vi "Registry FGV.vi"(7 "State (Get Logger)":T2(ring)=enum."Get Logger", 8 "error in (no error)":errorcluster, 9 "Debug Level in":T1, 10 "Sink(s)":refnum<class "Sink.lvclass">[](array[class]), 11 "Name":string) -> (0 "error out":errorcluster, 1 "Debug Level out":T1=enum."DEBUG", 2 "Sinks":refnum<class "Sink.lvclass">[](array[class]), 3 "Logger out":refnum<class "Logger.lvclass">)   [LabVIEW 2020, in "LV Log.lvlib"]
uses:
  LV Log.lvlib
  Logger/Logger.lvclass
  Sinks/Sink/Sink.lvclass
  Type Defs/Debug Level.ctl
  Registry/Registry.lvclass
  Registry/Registry.lvclass/Registry.ctl
  <vilib>/ErrorRing/Error Ring.xnode
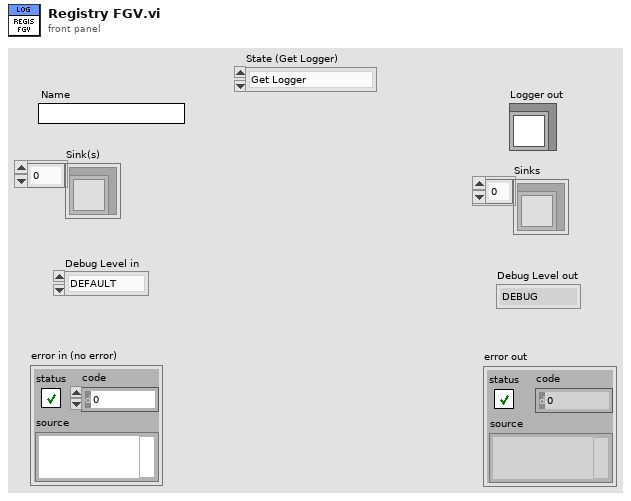
[diagram p1: front panel]
types:
  T1 = typedef "LV Log.lvlib/Debug Level.ctl" = enum16{"DEFAULT", "DEBUG", "INFO", "WARN", "ERROR", "FATAL"}
  T2 = enum16{"Init", "Get Logger", "Register Sink", "Set Global Debug Level", "Get Sinks", "Get Global Debug Level", "Register Logger"}
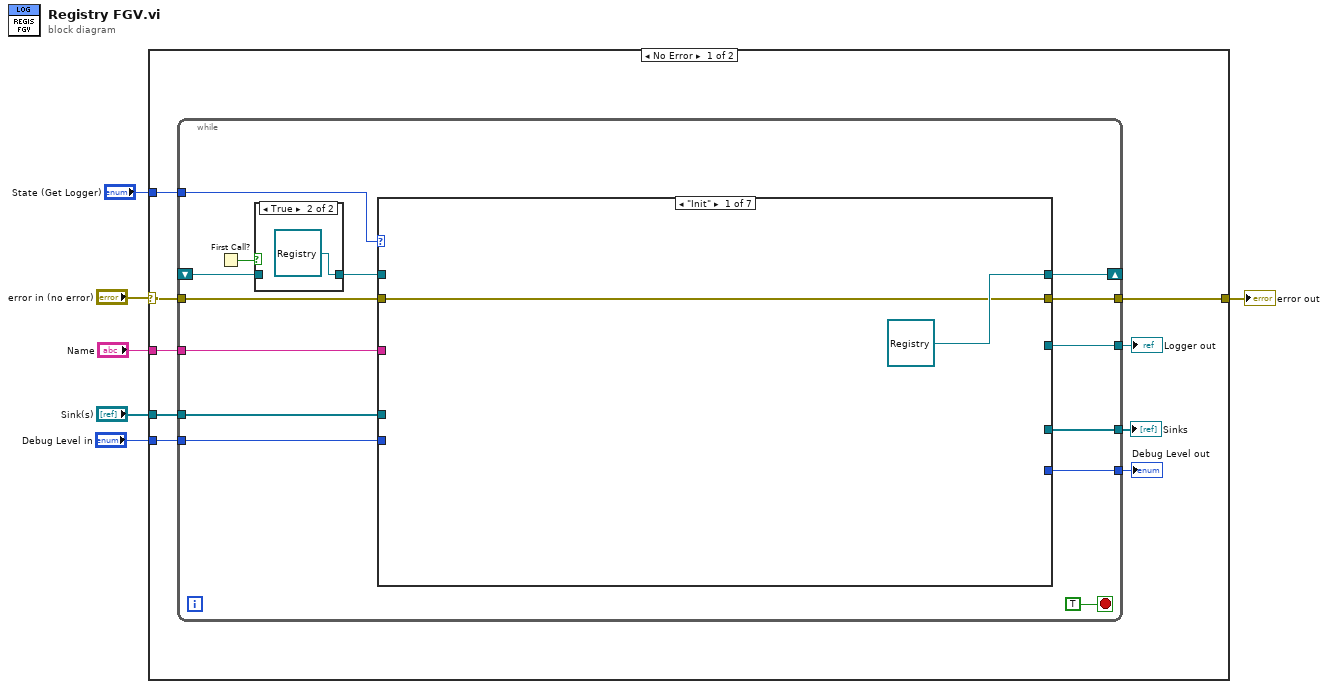
[diagram p0: block diagram]
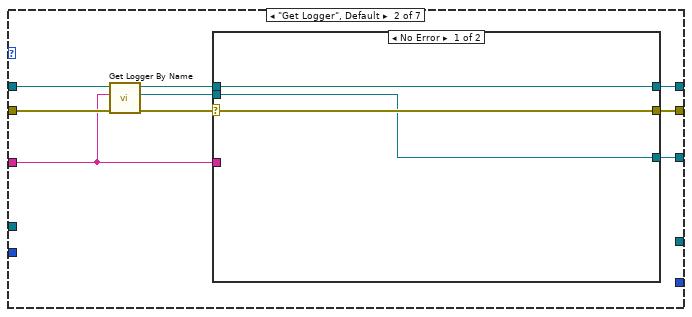
[diagram p3: hidden frame]
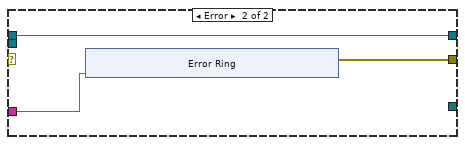
[diagram p4: hidden frame]
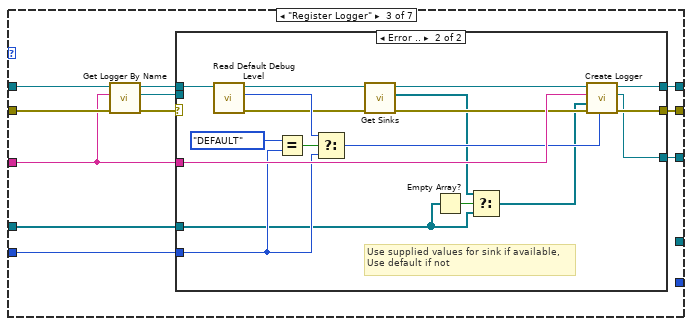
[diagram p5: hidden frame]
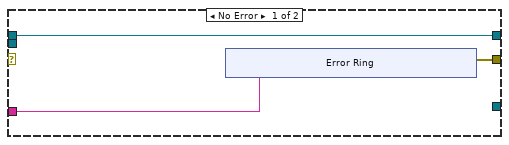
[diagram p6: hidden frame]
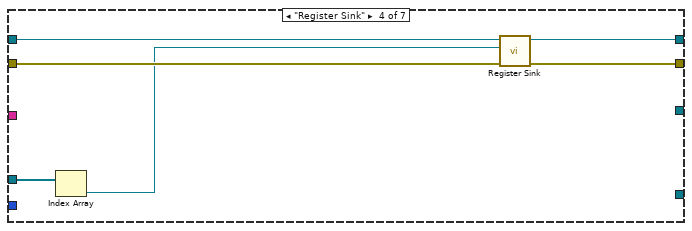
[diagram p7: hidden frame]
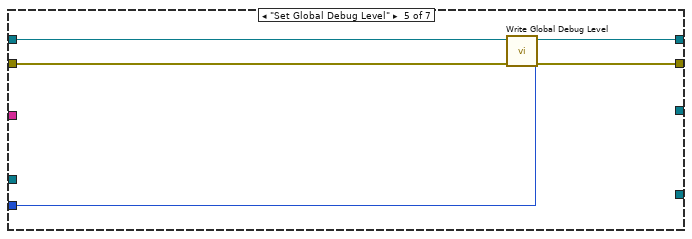
[diagram p8: hidden frame]
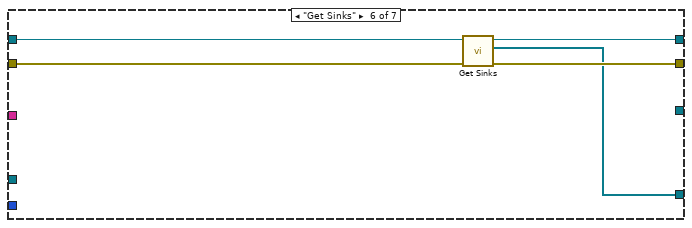
[diagram p9: hidden frame]
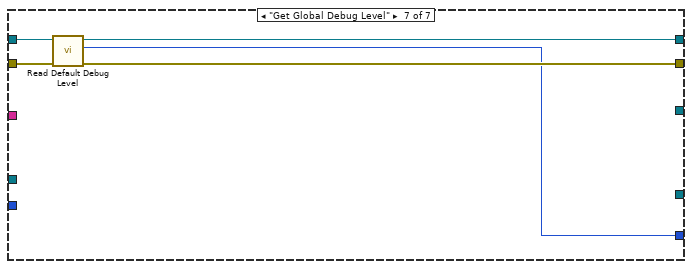
[diagram p10: hidden frame]
diagram:
  n1 = case shown="No Error" "error in (no error)" {
    selector: "error in (no error)" -> [w13 w112]
    tunnel: "State (Get Logger)" -> [w15 _]
    tunnel: "Name" -> [w14 _]
    tunnel: [w12 w112] -> w3
    tunnel: "Sink(s)" -> [w10 _]
    tunnel: "Debug Level in" -> [w8 _]
    frame No Error {
      n2 = while {
        shift-right: [w28] -> _
        shift-left: _ -> [w20]
        tunnel: w15 -> [w27]
        tunnel: w14 -> [w26]
        tunnel: w13 -> [w25]
        tunnel: [w24] -> w12
        tunnel: [w23] -> w11
        tunnel: w10 -> [w22]
        tunnel: [w21] -> w9
        tunnel: w8 -> [w17]
        tunnel: [w16] -> w7
        stop <- TRUE stop-if-true
        n3 = First Call?() -> (First Call?: T/F=w18:bool)
        n4 = case shown="True" w18 {
          tunnel: w20 -> [w30 _]
          tunnel: [w30 refnum<class "Registry.lvclass"> refnum ("LV Logging.lvlib:Registry.lvclass")] -> w19
          frame False {
          }
          frame True {
          }
        }
        n5 = case shown="\"Init\"" w27 {
          tunnel: [refnum<class "Registry.lvclass"> refnum ("LV Logging.lvlib:Registry.lvclass") w40 w62 w94 w100 w103 w109] -> w28
          tunnel: w26 -> [_ w35 w57 _ _ _ _]
          tunnel: w19 -> [_ w42 w64 w95 w101 w105 w111]
          tunnel: w25 -> [w32 w37 w59 w96 w99 w106 w110]
          tunnel: [w32 w36 w58 w93 w98 w104 w108] -> w24
          tunnel: [_ w34 w56 _ _ _ _] -> w23
          tunnel: w22 -> [_ _ w55 w92 _ _ _]
          tunnel: [_ _ _ _ _ w102 _] -> w21
          tunnel: w17 -> [_ _ w54 _ w97 _ _]
          tunnel: [_ _ _ _ _ _ w107] -> w16
          frame "Init" {
          }
          frame "Get Logger", Default {
            n6 = call "Get Logger By Name.vi"("error in (no error)"=w37, "Name"=w35, "Registry in"=w42) -> ("error out"=w39:errorcluster, "Logger"=w38:refnum<class "Logger.lvclass">, "Registry out"=w41:refnum<class "Registry.lvclass">)  [unwired: 6 in]
            n7 = case shown="No Error" w39 {
              selector: w39 -> [w44 _]
              tunnel: w41 -> [w45 w48]
              tunnel: [w45 w48] -> w40
              tunnel: w38 -> [w43 _]
              tunnel: [w44 w47] -> w36
              tunnel: w35 -> [_ w46]
              tunnel: [w43 _] -> w34
              frame No Error {
              }
              frame Error {
                n8 = xnode "Error Ring"("parameter 0"=w46) -> ("error out"=w47:errorcluster)
              }
            }
          }
          frame "Register Logger" {
            n9 = call "Get Logger By Name.vi"("error in (no error)"=w59, "Name"=w57, "Registry in"=w64) -> ("error out"=w61:errorcluster, "Logger"=w60:refnum<class "Logger.lvclass">, "Registry out"=w63:refnum<class "Registry.lvclass">)  [unwired: 6 in]
            n10 = case shown="Error .." w61 {
              tunnel: w63 -> [w67 w82]
              tunnel: [w67 w90] -> w62
              tunnel: w60 -> [_ _]
              tunnel: [w66 w89] -> w58
              tunnel: w57 -> [w65 w88]
              tunnel: [_ w87] -> w56
              tunnel: w55 -> [_ w74]
              tunnel: w54 -> [_ w84]
              frame No Error {
                n11 = xnode "Error Ring"("parameter 0"=w65) -> ("error out"=w66:errorcluster)
              }
              frame Error {
                # "Use supplied values for sink if available,\nUse default if not"
                n12 = call "Read Default Debug Level.vi"("Registry in"=w82) -> ("error out"=w78:errorcluster, "Debug Level"=w81:T1, "Registry out"=w80:refnum<class "Registry.lvclass">)  [unwired: 8 in]
                n13 = Equal?(x=Debug_Level."DEFAULT", y=w84) -> (x = y?=w85:bool)
                n14 = Select(t=w81, s=w85, f=w84) -> (s? t:f=w83:T1)
                n15 = call "Get Sinks.vi"("error in (no error)"=w78, "Registry in"=w80) -> ("error out"=w77:errorcluster, "Sinks"=w75:refnum<class "Sink.lvclass">[], "Registry out"=w79:refnum<class "Registry.lvclass">)  [unwired: 7 in]
                n16 = Empty Array?(array=w74) -> (empty?=w76:bool)
                n17 = Select(t=w75, s=w76, f=w74) -> (s? t:f=w73:refnum<class "Sink.lvclass">[])
                n18 = call "Create Logger.vi"("Debug Level"=w83, "error in (no error)"=w77, "Sinks"=w73, "Name"=w88, "Registry in"=w79) -> ("error out"=w89:errorcluster, "Logger out"=w87:refnum<class "Logger.lvclass">, "Registry out"=w90:refnum<class "Registry.lvclass">)  [unwired: 4 in]
              }
            }
          }
          frame "Register Sink" {
            n19 = Index Array(array=w92) -> (element=w91:refnum<class "Sink.lvclass">)  [unwired: 1 in]
            n20 = call "Register Sink.vi"("error in (no error)"=w96, "Sink"=w91, "Registry in"=w95) -> ("error out"=w93:errorcluster, "Registry out"=w94:refnum<class "Registry.lvclass">)  [unwired: 7 in]
          }
          frame "Set Global Debug Level" {
            n21 = call "Write Global Debug Level.vi"("error in (no error)"=w99, "Debug Level"=w97, "Registry in"=w101) -> ("error out"=w98:errorcluster, "Registry out"=w100:refnum<class "Registry.lvclass">)  [unwired: 7 in]
          }
          frame "Get Sinks" {
            n22 = call "Get Sinks.vi"("error in (no error)"=w106, "Registry in"=w105) -> ("error out"=w104:errorcluster, "Sinks"=w102:refnum<class "Sink.lvclass">[], "Registry out"=w103:refnum<class "Registry.lvclass">)  [unwired: 7 in]
          }
          frame "Get Global Debug Level" {
            n23 = call "Read Default Debug Level.vi"("error in (no error)"=w110, "Registry in"=w111) -> ("error out"=w108:errorcluster, "Debug Level"=w107:T1, "Registry out"=w109:refnum<class "Registry.lvclass">)  [unwired: 7 in]
          }
        }
      }
      "Logger out" <- w11
      "Sinks" <- w9
      "Debug Level out" <- w7
    }
    frame Error {
    }
  }
  "error out" <- w3
